vi "流量计UI.vi"() -> ()   [LabVIEW 2016]
uses:
  <vilib>/Plasmionique/MB Master/MB_Master_Serial/MB_Master_Serial.lvclass
  D:/Program Files (x86)/National Instruments/LabVIEW 2016/vi.lib/Plasmionique/MB Master/MB_Master/MB_Master.lvclass
  <vilib>/Analysis/baseanly.llb/Mean (DBL).vi
  <vilib>/Utility/config.llb/NI_LVConfig.lvlib
  <vilib>/Analysis/NI_AALBase.lvlib
panel:
  out "平均水位":dbl
  out "总累积流量":dbl
  out "平均流速":dbl
  out "总流量":dbl
  in  "选项卡控件":enum32{"LDM51", "MGG/KL QC", "斯坦道功率测流"}(tab)
  out "数组":T1[](array[typedef])
  out "数组 2":T2[](array[typedef]) {"累积流量单位" items=["L", "M3", "T", "USG"]; "瞬时流量单位" items=["L/S", "L/M", "L/H", "M3/S", "M3/M", "M3/H", "T/S", "T/M", "T/H", "GPS", "GPM", "GPH"]}
  out "数组 3":T5[](array[typedef])
  out "MB_Serial session":refnum<class "MB_Master_Serial.lvclass">
  in  "斯坦道功率测流":bool
  in  "流量计启用 3":bool
  in  "数量 3":u16
  out "流量计类型 3":T6=enum."斯坦道功率测流"
  in  "流量计启用 2":bool
  in  "数量 2":u16
  out "流量计类型 2":T6=enum."MGG/KL QC"
  in  "数量":u16
  out "流量计类型":T6
  in  "流量计启用":bool
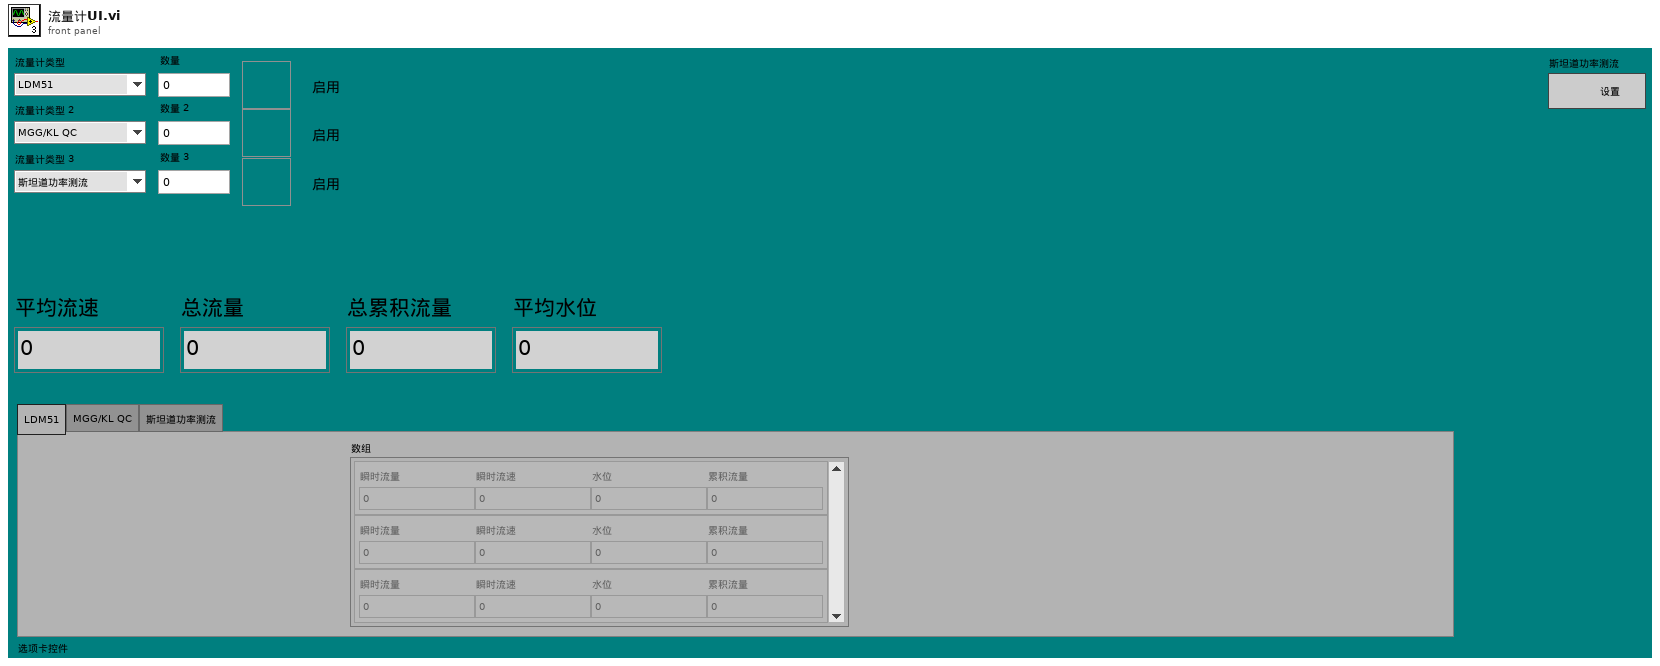
[diagram p1: front panel]
types:
  T1 = typedef "LDM51明渠流量计.lvlib/读取值.ctl" = cluster{"瞬时流量":sgl, "瞬时流速":sgl, "水位":sgl, "累积流量":sgl}
  T2 = typedef "MGG-KL-QC流量计.lvlib/读取值.ctl" = cluster{"瞬时流量":sgl, "瞬时流速":sgl, "流量百分比":sgl, "流体电导比":sgl, "正向累积数值":sgl, "反向累积数值":sgl, "瞬时流量单位":T3, "累积流量单位":T4, "上限报警":u16, "下限报警":u16, "空管报警":u16, "系统报警":u16}
  T3 = typedef "MGG-KL-QC流量计.lvlib/瞬时流量单位.ctl" = u16
  T4 = typedef "MGG-KL-QC流量计.lvlib/累积流量单位.ctl" = u16
  T5 = typedef "斯坦道功率测流.lvlib/状态值.ctl" = cluster{"1号瞬时流量":dbl, "2号瞬时流量":dbl, "3号瞬时流量":dbl, "4号瞬时流量":dbl, "5号瞬时流量":dbl, "6号瞬时流量":dbl, "1号累积流量":dbl, "2号累积流量":dbl, "3号累积流量":dbl, "4号累积流量":dbl, "5号累积流量":dbl, "6号累积流量":dbl, "总瞬时流量":dbl, "总累积流量":dbl}
  T6 = typedef "流量计类型.ctl" = enum16{"LDM51", "MGG/KL QC", "斯坦道功率测流", "WL-1A1"}
  T7 = cluster{"时间标识":timestamp, "测量模式":string, "数据类型":string, "监测值":sgl, "单位":string, "数据标识":string, "因子编码":string}
  T8 = typedef "LVDateTimeRec.ctl" = cluster{"秒数的小数部分":dbl, "秒":i32, "分":i32, "时":i32, "日":i32, "月":i32, "年":i32, "天数（周）":i32, "天数（年）":i32, "DST":i32}
  T9 = typedef "NI_LVConfig.lvlib/Config Data RefNum.ctl" = refnum<k1>
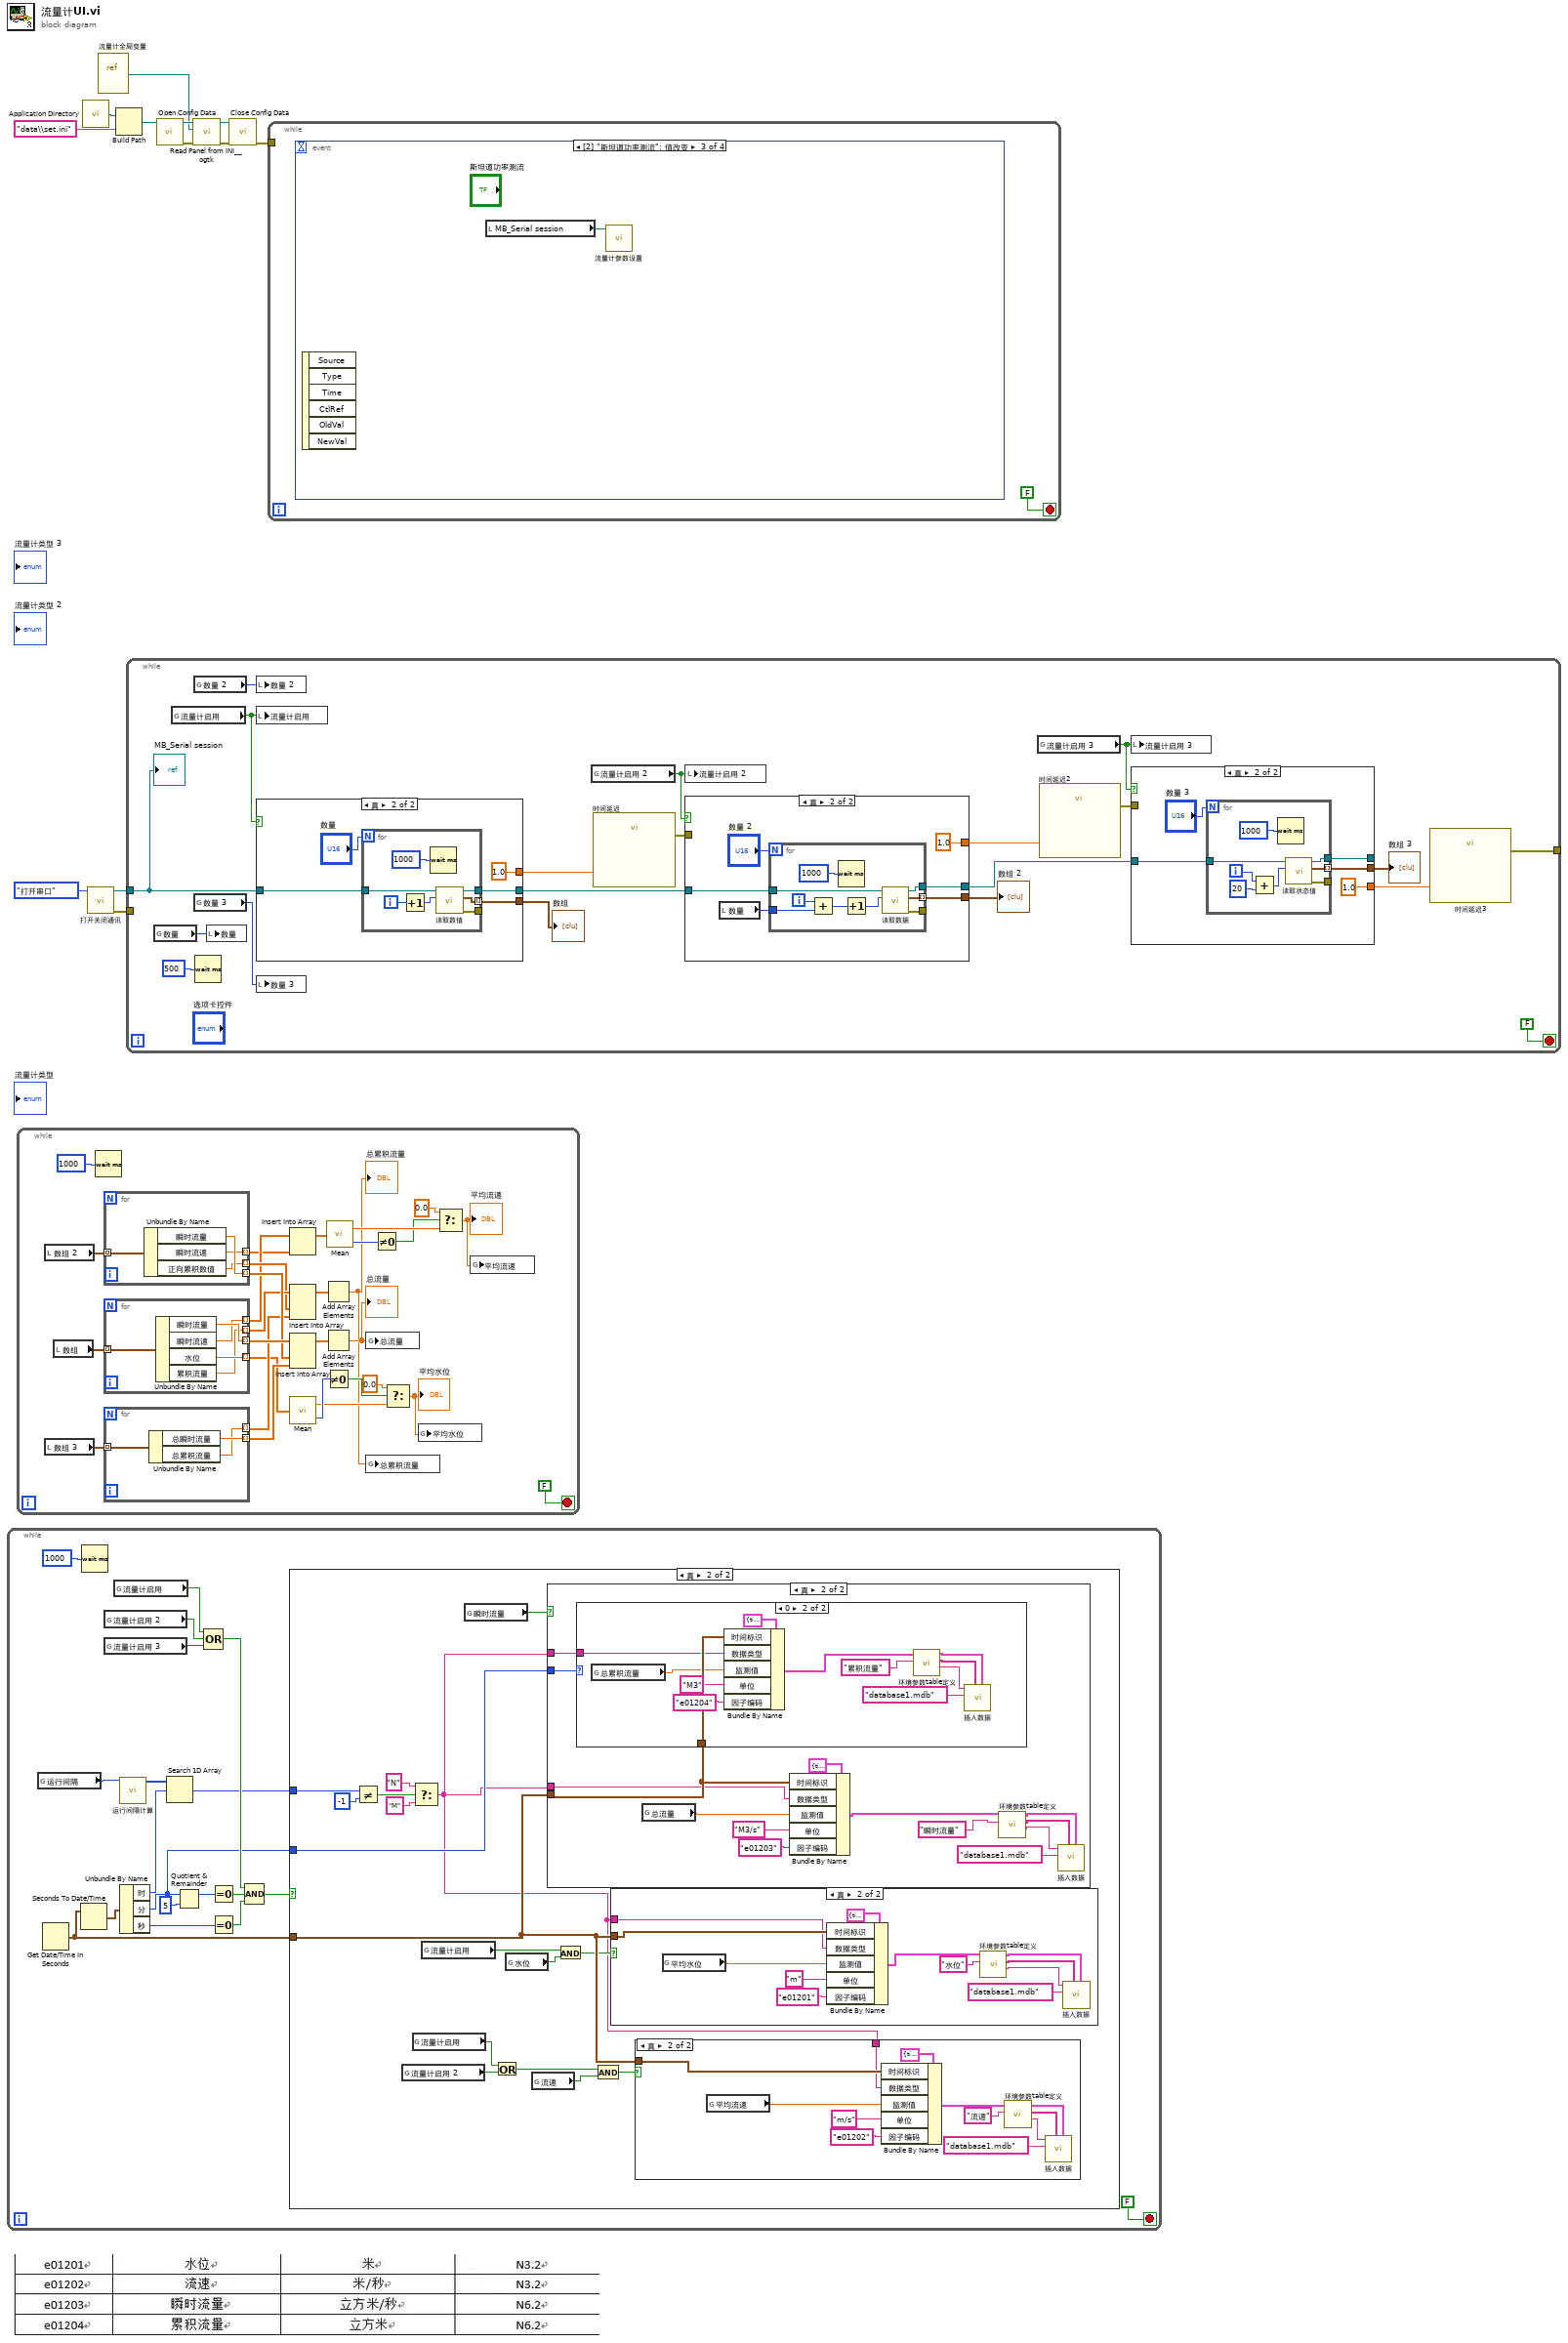
[diagram p0: block diagram]
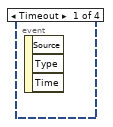
[diagram p7: hidden frame]
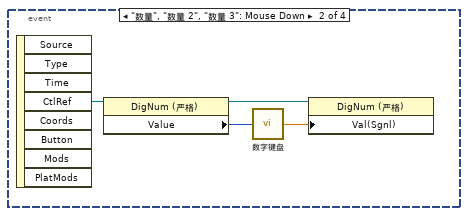
[diagram p8: hidden frame]
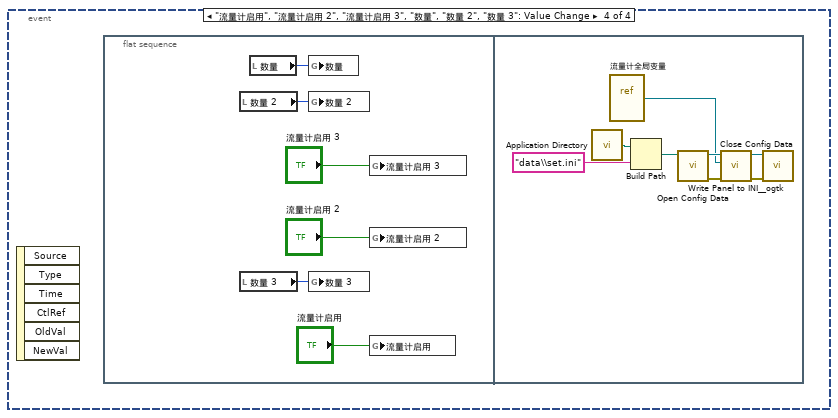
[diagram p9: hidden frame]
diagram:
  n1 = while {
    stop <- FALSE stop-if-true
    n2 = global read "流量计全局变量.vi" "运行间隔"() -> (w13:i16)
    n3 = Get Date/Time In Seconds() -> (seconds since 1Jan1904=w30:timestamp)
    n4 = Seconds To Date/Time(time stamp (now)=w30) -> (date time rec=w29:T8)  [unwired: 1 in]
    n5 = Wait (ms)(milliseconds to wait=u32 1000 ("等待时间（毫秒）")) -> ()  [unwired: 1 out]
    n6 = global read "流量计全局变量.vi" "流量计启用 2"() -> (w20:bool)
    n7 = global read "流量计全局变量.vi" "流量计启用 3"() -> (w19:bool)
    n8 = global read "流量计全局变量.vi" "流量计启用"() -> (w21:bool)
    n9 = call "运行间隔计算.vi"("运行周期"=w13) -> ("数组"=w16:i32[])  [unwired: 10 in]
    n10 = Unbundle By Name(w29) -> ("时"=w17:i32, "分"=w14:i32, "秒"=w27:i32)
    n11 = Search 1D Array(1D array=w16, element=w17) -> (index of element=w15:i32)  [unwired: 1 in]
    n12 = Quotient & Remainder(x=w14, y=5) -> (x-y*floor(x/y)=w26:i32)  [unwired: 1 out]
    n13 = Compound Arithmetic op=OR ("复合运算")(w21, w20, w19) -> (w18:bool)
    n14 = Equal To 0?(x=w26) -> (x = 0?=w25:bool)
    n15 = Equal To 0?(x=w27) -> (x = 0?=w24:bool)
    n16 = Compound Arithmetic op=AND ("复合运算")(w18, w25, w24) -> (w23:bool)
    n17 = case shown="真" w23 {
      tunnel: w30 -> [_ w47]
      tunnel: w15 -> [_ w34]
      tunnel: w14 -> [_ w33]
      frame False {
      }
      frame True {
        n18 = Not Equal?(x=w34, y=-1) -> (x != y?=w37:bool)
        n19 = global read "流量计全局变量.vi" "流量计启用 2"() -> (w39:bool)
        n20 = global read "流量计全局变量.vi" "流量计启用"() -> (w40:bool)
        n21 = Select(t="N" ("单位"), s=w37, f="M" ("单位")) -> (s? t:f=w32:string)
        n22 = global read "流量计全局变量.vi" "流量计启用"() -> (w45:bool)
        n23 = global read "副屏设置全局变量.vi" "瞬时流量"() -> (w48:bool)
        n24 = Or(x=w40, y=w39) -> (x .or. y?=w41:bool)
        n25 = global read "副屏设置全局变量.vi" "水位"() -> (w46:bool)
        n26 = global read "副屏设置全局变量.vi" "流速"() -> (w43:bool)
        n27 = case shown="真" w48 {
          tunnel: w47 -> [_ w69]
          tunnel: w32 -> [_ w73]
          tunnel: w33 -> [_ w72]
          tunnel: w32 -> [_ w67]
          frame False {
          }
          frame True {
            n28 = case shown="0" w72 {
              tunnel: w69 -> [_ w85]
              tunnel: w73 -> [_ w82]
              frame Default {
              }
              frame 0 {
                n29 = global read "流量计全局变量.vi" "总累积流量"() -> (w83:dbl)
                n30 = Bundle By Name(cluster=T7 {"时间标识"=timestamp(0 s since 1904-01-01), "测量模式"="水样测试", "数据类型"="N", "监测值"=0.0, "单位"="mg/L", "数据标识"="N", "因子编码"=""} ("data"), "时间标识"=w85, "数据类型"=w82, "监测值"=w83, "单位"="M3", "因子编码"="e01204") -> (w79:T7)
                n31 = call "环境参数table定义.vi"("table 输入"="累积流量", "data"=w79) -> ("table 输出"=w75:string, "columns"=w76:string[], "data输出"=w77:T7)  [unwired: 7 in]
                n32 = call "插入数据.vi"("data"=w77, "columns"=w76, "database"="database1.mdb" ("table 输入"), "table"=w75) -> ()  [unwired: 7 in, 1 out]
              }
            }
            n33 = global read "流量计全局变量.vi" "总流量"() -> (w68:dbl)
            n34 = Bundle By Name(cluster=T7 {"时间标识"=timestamp(0 s since 1904-01-01), "测量模式"="水样测试", "数据类型"="N", "监测值"=0.0, "单位"="mg/L", "数据标识"="N", "因子编码"=""} ("data"), "时间标识"=w69, "数据类型"=w67, "监测值"=w68, "单位"="M3/s", "因子编码"="e01203") -> (w65:T7)
            n35 = call "环境参数table定义.vi"("table 输入"="瞬时流量", "data"=w65) -> ("table 输出"=w61:string, "columns"=w62:string[], "data输出"=w63:T7)  [unwired: 7 in]
            n36 = call "插入数据.vi"("data"=w63, "columns"=w62, "database"="database1.mdb" ("table 输入"), "table"=w61) -> ()  [unwired: 7 in, 1 out]
          }
        }
        n37 = And(x=w45, y=w46) -> (x .and. y?=w44:bool)
        n38 = And(x=w41, y=w43) -> (x .and. y?=w42:bool)
        n39 = case shown="真" w44 {
          tunnel: w47 -> [_ w56]
          tunnel: w32 -> [_ w55]
          frame False {
          }
          frame True {
            n40 = global read "流量计全局变量.vi" "平均水位"() -> (w54:dbl)
            n41 = Bundle By Name(cluster=T7 {"时间标识"=timestamp(0 s since 1904-01-01), "测量模式"="水样测试", "数据类型"="N", "监测值"=0.0, "单位"="mg/L", "数据标识"="N", "因子编码"=""} ("data"), "时间标识"=w56, "数据类型"=w55, "监测值"=w54, "单位"="m", "因子编码"="e01201") -> (w50:T7)
            n42 = call "环境参数table定义.vi"("table 输入"="水位", "data"=w50) -> ("table 输出"=w51:string, "columns"=w52:string[], "data输出"=w53:T7)  [unwired: 7 in]
            n43 = call "插入数据.vi"("data"=w53, "columns"=w52, "database"="database1.mdb" ("table 输入"), "table"=w51) -> ()  [unwired: 7 in, 1 out]
          }
        }
        n44 = case shown="真" w42 {
          tunnel: w47 -> [_ w93]
          tunnel: w32 -> [_ w92]
          frame False {
          }
          frame True {
            n45 = global read "流量计全局变量.vi" "平均流速"() -> (w94:dbl)
            n46 = Bundle By Name(cluster=T7 {"时间标识"=timestamp(0 s since 1904-01-01), "测量模式"="水样测试", "数据类型"="N", "监测值"=0.0, "单位"="mg/L", "数据标识"="N", "因子编码"=""} ("data"), "时间标识"=w93, "数据类型"=w92, "监测值"=w94, "单位"="m/s", "因子编码"="e01202") -> (w90:T7)
            n47 = call "环境参数table定义.vi"("table 输入"="流速", "data"=w90) -> ("table 输出"=w87:string, "columns"=w88:string[], "data输出"=w89:T7)  [unwired: 7 in]
            n48 = call "插入数据.vi"("data"=w89, "columns"=w88, "database"="database1.mdb" ("table 输入"), "table"=w87) -> ()  [unwired: 7 in, 1 out]
          }
        }
      }
    }
  }
  n49 = while {
    stop <- FALSE stop-if-true
    n50 = local read "数组 2"() -> (w124:T2[])
    n51 = local read "数组 3"() -> (w123:T5[])
    n52 = local read "数组"() -> (w127:T1[])
    n53 = Wait (ms)(milliseconds to wait=u32 1000 ("等待时间（毫秒）")) -> ()  [unwired: 1 out]
    n54 = for {
      tunnel: w124 -> [w134] mode=indexing
      tunnel: [w133] -> w121 mode=indexing
      tunnel: [w132] -> w113 mode=indexing
      tunnel: [w131] -> w118 mode=indexing
      n55 = Unbundle By Name(w134) -> ("瞬时流量"=w133:sgl, "瞬时流速"=w132:sgl, "正向累积数值"=w131:sgl)
    }
    n56 = for {
      tunnel: w127 -> [w139] mode=indexing
      tunnel: [w138] -> w122 mode=indexing
      tunnel: [w137] -> w114 mode=indexing
      tunnel: [w136] -> w103 mode=indexing
      tunnel: [w135] -> w119 mode=indexing
      n57 = Unbundle By Name(w139) -> ("瞬时流量"=w138:sgl, "瞬时流速"=w137:sgl, "水位"=w136:sgl, "累积流量"=w135:sgl)
    }
    n58 = for {
      tunnel: w123 -> [w130] mode=indexing
      tunnel: [w129] -> w120 mode=indexing
      tunnel: [w128] -> w117 mode=indexing
      n59 = Unbundle By Name(w130) -> ("总瞬时流量"=w129:dbl, "总累积流量"=w128:dbl)
    }
    n60 = Insert Into Array(array=w114, new element=w113) -> (w108:sgl[])  [unwired: 1 in]
    n61 = Insert Into Array(array=w119, new element #1=w118, new element #2=w117) -> (w115:sgl[])  [unwired: 1 in]
    n62 = Insert Into Array(array=w122, new element #1=w121, new element #2=w120) -> (w116:sgl[])  [unwired: 1 in]
    n63 = call-poly <vilib>:"Mean.vi"("X"=w103) -> ("mean"=w104:dbl, "error"=w107:i32)
    n64 = Add Array Elements(numeric array=w115) -> (sum=w100:sgl)
    "总累积流量" <- w100
    n65 = Add Array Elements(numeric array=w116) -> (sum=w102:sgl)
    "总流量" <- w102
    n66 = Not Equal To 0?(x=w107) -> (x != 0?=w106:bool)
    n67 = call-poly <vilib>:"Mean.vi"("X"=w108) -> ("mean"=w112:dbl, "error"=w109:i32)
    n68 = global write "流量计全局变量.vi" "总流量"(w102) -> ()
    n69 = global write "流量计全局变量.vi" "总累积流量"(w100) -> ()
    n70 = Not Equal To 0?(x=w109) -> (x != 0?=w110:bool)
    n71 = Select(t=0.0, s=w106, f=w104) -> (s? t:f=w99:dbl)
    "平均水位" <- w99
    n72 = global write "流量计全局变量.vi" "平均水位"(w99) -> ()
    n73 = Select(t=0.0, s=w110, f=w112) -> (s? t:f=w101:dbl)
    "平均流速" <- w101
    n74 = global write "流量计全局变量.vi" "平均流速"(w101) -> ()
  }
  n75 = call <vilib>:"Application Directory.vi"() -> ("Application Directory"=w10:path)
  n76 = call "打开关闭通讯.vi"("功能输入"=enum16{"打开串口", "关闭串口"}."打开串口") -> ("error out"=w3:errorcluster, "MB_Serial session"=w2:refnum<class "MB_Master_Serial.lvclass">)  [unwired: 9 in]
  n77 = vi-ref "流量计全局变量.vi"() -> (w1:refnum<vi>)
  n78 = Build Path(base path=w10, name or relative path="data\\set.ini" ("名称或相对路径")) -> (appended path=w11:path)
  n79 = while {
    tunnel: w3 -> [_]
    tunnel: w2 -> [w149]
    tunnel: [w140] -> _
    stop <- FALSE stop-if-true
    n80 = global read "流量计全局变量.vi" "数量"() -> (w148:u16)
    n81 = global read "流量计全局变量.vi" "流量计启用"() -> (w157:bool)
    n82 = global read "流量计全局变量.vi" "数量 2"() -> (w147:u16)
    n83 = global read "流量计全局变量.vi" "数量 3"() -> (w146:u16)
    n84 = Wait (ms)(milliseconds to wait=u32 500 ("等待时间（毫秒）")) -> ()  [unwired: 1 out]
    n85 = local write "数量"(w148) -> ()
    n86 = local write "数量 2"(w147) -> ()
    n87 = local write "流量计启用"(w157) -> ()
    n88 = case shown="真" w157 {
      tunnel: w149 -> [w190 w195]
      tunnel: [w190 w193] -> w156
      tunnel: [_ w192] -> w154
      tunnel: [_ 1.0 ("Delay Time (s)")] -> w145
      frame False {
      }
      frame True {
        n89 = for {
          N: "数量" -> [_]
          tunnel: w195 -> [w202]
          tunnel: [w201] -> _
          tunnel: [w198] -> w193
          tunnel: [w197] -> w192 mode=indexing
          i -> [w200]
          n90 = Increment(x=w200) -> (x+1=w199:i32)
          n91 = Wait (ms)(milliseconds to wait=u32 1000 ("等待时间（毫秒）")) -> ()  [unwired: 1 out]
          n92 = call "读取数值.vi"("Slave ID"=w199, "MB session in"=w202) -> ("error out"=w201:errorcluster, "读取值"=w197:T1, "MB session out"=w198:refnum<class "MB_Master_Serial.lvclass">)  [unwired: 7 in]
        }
      }
    }
    "数组" <- w154
    n93 = local write "数量 3"(w146) -> ()
    n94 = global read "流量计全局变量.vi" "流量计启用 2"() -> (w155:bool)
    n95 = call "时间延迟"("Delay Time (s)"=w145) -> ("error out"=w144:errorcluster)  [unwired: 10 in]
    n96 = local write "流量计启用 2"(w155) -> ()
    n97 = case shown="真" w155 {
      tunnel: w156 -> [w174 w179]
      tunnel: [w174 w177] -> w152
      tunnel: [_ w176] -> w153
      tunnel: w144 -> [_ _]
      tunnel: [_ 1.0 ("Delay Time (s)")] -> w143
      frame False {
      }
      frame True {
        n98 = local read "数量"() -> (w178:u16)
        n99 = for {
          N: "数量 2" -> [_]
          tunnel: w179 -> [w188]
          tunnel: w178 -> [w185]
          tunnel: [w184] -> w177
          tunnel: [w183] -> w176 mode=indexing
          tunnel: [w182] -> _
          i -> [w186]
          n100 = Add(x=w186, y=w185) -> (x+y=w187:i32)
          n101 = Wait (ms)(milliseconds to wait=u32 1000 ("等待时间（毫秒）")) -> ()  [unwired: 1 out]
          n102 = Increment(x=w187) -> (x+1=w189:i32)
          n103 = call "读取数据.vi"("Slave ID"=w189, "MB session in"=w188) -> ("error out"=w182:errorcluster, "读取值"=w183:T2, "MB session out"=w184:refnum<class "MB_Master_Serial.lvclass">)  [unwired: 6 in, 1 out]
        }
      }
    }
    "数组 2" <- w153
    n104 = global read "流量计全局变量.vi" "流量计启用 3"() -> (w151:bool)
    n105 = call "时间延迟2"("Delay Time (s)"=w143) -> ("error out"=w141:errorcluster)  [unwired: 10 in]
    n106 = local write "流量计启用 3"(w151) -> ()
    n107 = case shown="真" w151 {
      tunnel: w152 -> [w160 w165]
      tunnel: [w160 w164] -> _
      tunnel: [_ w162] -> w150
      tunnel: [_ 1.0 ("Delay Time (s)")] -> w142
      tunnel: w141 -> [_ _]
      frame False {
      }
      frame True {
        n108 = for {
          N: "数量 3" -> [_]
          tunnel: w165 -> [w171]
          tunnel: [w168] -> w164
          tunnel: [w169] -> _
          tunnel: [w167] -> w162 mode=indexing
          i -> [w173]
          n109 = Add(x=w173, y=20) -> (x+y=w170:i32)
          n110 = Wait (ms)(milliseconds to wait=u32 1000 ("等待时间（毫秒）")) -> ()  [unwired: 1 out]
          n111 = call "读取状态值.vi"("Slave ID"=w170, "MB session in"=w171) -> ("error out"=w169:errorcluster, "状态值"=w167:T5, "MB session out"=w168:refnum<class "MB_Master_Serial.lvclass">)  [unwired: 6 in, 1 out]
        }
      }
    }
    "数组 3" <- w150
    n112 = call "时间延迟3"("Delay Time (s)"=w142) -> ("error out"=w140:errorcluster)  [unwired: 10 in]
    "MB_Serial session" <- w149
  }
  n113 = call <vilib>:"Open Config Data.vi"("configuration file path"=w11) -> ("error out"=w8:errorcluster, "refnum"=w9:T9)  [unwired: 8 in, 1 out]
  n114 = call <userlib>:"Read Panel from INI__ogtk.vi"("error in (no error)"=w8, "VI ref"=w1, "refnum"=w9) -> ("error out"=w6:errorcluster, "refnum out"=w7:T9)  [unwired: 7 in]
  n115 = call <vilib>:"Close Config Data.vi"("error in (no error)"=w6, "refnum"=w7) -> ("error out"=w5:errorcluster)  [unwired: 8 in, 1 out]
  n116 = while {
    tunnel: w5 -> [_]
    stop <- FALSE stop-if-true
    n117 = event shown="[2] \"斯坦道功率测流\": 值改变" {
      selector: _ -> [_ _ _ _]
      dyn-events: _ -> [_ _ _ _]
      timeout: _ -> [_ _ _ _]
      event Timeout {
        n118 = event-data() -> ()  [unwired: 1 in, 3 out]
      }
      event "数量", "数量 2", "数量 3": Mouse Down {
        n119 = event-data() -> ("CtlRef"=w207:refnum<vi>)  [unwired: 1 in, 7 out]
        n120 = property class="DigNum (严格)"(reference=w207) -> (reference out=w205:refnum<vi>, "Value"=w206:u16)  [unwired: 1 in, 1 out]
        n121 = call "数字键盘.vi"("OldNumber"=w206) -> ("NewNumber"=w204:sgl)
        n122 = property class="DigNum (严格)"(reference=w205, "Val(Sgnl)"=w204) -> ()  [unwired: 1 in, 2 out]
      }
      event "斯坦道功率测流": Value Change {
        n123 = event-data() -> ()  [unwired: 1 in, 6 out]
        n124 = local read "MB_Serial session"() -> (w208:refnum<class "MB_Master_Serial.lvclass">)
        n125 = call "流量计参数设置.vi"("MB session in"=w208) -> ()  [unwired: 11 in]
      }
      event "流量计启用", "流量计启用 2", "流量计启用 3", "数量", "数量 2", "数量 3": Value Change {
        n126 = event-data() -> ()  [unwired: 1 in, 6 out]
        n127 = flat-sequence {
          frame #0 {
            n128 = local read "数量 2"() -> (w210:u16)
            n129 = local read "数量 3"() -> (w209:u16)
            n130 = local read "数量"() -> (w211:u16)
            n131 = global write "流量计全局变量.vi" "数量"(w211) -> ()
            n132 = global write "流量计全局变量.vi" "数量 2"(w210) -> ()
            n133 = global write "流量计全局变量.vi" "数量 3"(w209) -> ()
            n134 = global write "流量计全局变量.vi" "流量计启用 3"("流量计启用 3") -> ()
            n135 = global write "流量计全局变量.vi" "流量计启用 2"("流量计启用 2") -> ()
            n136 = global write "流量计全局变量.vi" "流量计启用"("流量计启用") -> ()
          }
          frame #1 {
            n137 = call <vilib>:"Application Directory.vi"() -> ("Application Directory"=w218:path)
            n138 = vi-ref "流量计全局变量.vi"() -> (w215:refnum<vi>)
            n139 = Build Path(base path=w218, name or relative path="data\\set.ini" ("名称或相对路径")) -> (appended path=w217:path)
            n140 = call <vilib>:"Open Config Data.vi"("configuration file path"=w217) -> ("error out"=w220:errorcluster, "refnum"=w222:T9)  [unwired: 8 in, 1 out]
            n141 = call <userlib>:"Write Panel to INI__ogtk.vi"("error in (no error)"=w220, "VI ref"=w215, "refnum"=w222) -> ("error out"=w219:errorcluster, "refnum out"=w221:T9)  [unwired: 7 in]
            n142 = call <vilib>:"Close Config Data.vi"("error in (no error)"=w219, "refnum"=w221) -> ()  [unwired: 8 in, 2 out]
          }
        }
      }
    }
  }
